vi "createfolderincrementing.vi"(8 "error in (no error)":errorcluster, 10 "Base path":path=path "bttt", 11 "Folder Name":string) -> (0 "error out":errorcluster, 3 "created path":path)   [LabVIEW 2017]
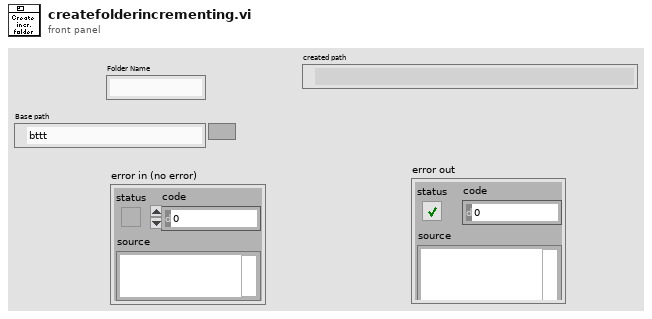
[diagram p1: front panel]
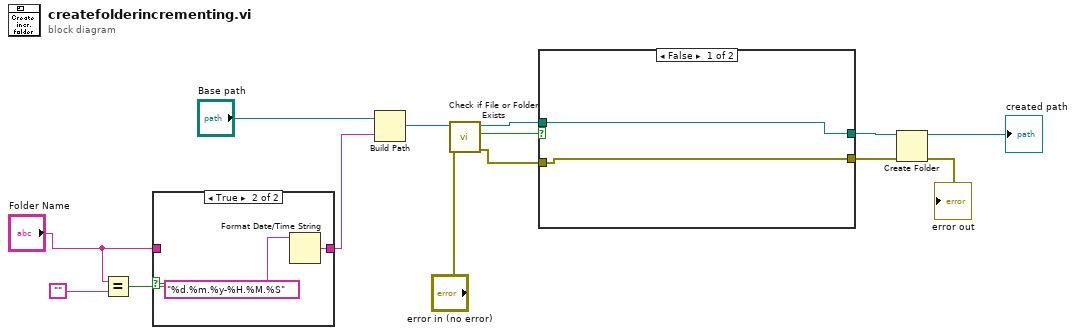
[diagram p0: block diagram]
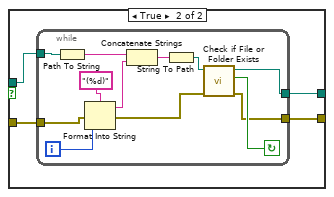
[diagram p3: hidden frame]
diagram:
  n1 = Equal?(x="Folder Name", y="") -> (x = y?=w4:bool)
  n2 = case shown="True" w4 {
    tunnel: [w15 w17] -> w3
    tunnel: "Folder Name" -> [w15 _]
    frame False {
    }
    frame True {
      n3 = Format Date/Time String(time format string (%c)="%d.%m.%y-%H.%M.%S") -> (date/time string=w17:string)  [unwired: 2 in]
    }
  }
  n4 = Build Path(base path="Base path", name or relative path=w3) -> (appended path=w14:path)
  n5 = call <vilib>:"Check if File or Folder Exists.vi"("error in (no error)"="error in (no error)", "path"=w14) -> ("error out"=w8:errorcluster, "file or folder exists?"=w13:bool, "dup path"=w11:path)  [unwired: 7 in]
  n6 = case shown="False" w13 {
    tunnel: [w19 w22] -> w12
    tunnel: w11 -> [w19 w23]
    tunnel: [w18 w21] -> w9
    tunnel: w8 -> [w18 w20]
    frame False {
    }
    frame True {
      n7 = while {
        tunnel: w23 -> [w28]
        tunnel: [w32] -> w22
        tunnel: [w31] -> w21
        tunnel: w20 -> [w29]
        i -> [w34]
        stop <- w35 continue-if-true
        n8 = Path To String(path=w28) -> (string=w27:string)
        n9 = Format Into String(format string="(%d)", error in=w29, w34) -> (resulting string=w26:string, error out=w30:errorcluster)  [unwired: 1 in]
        n10 = Concatenate Strings(w27, w26) -> (w25:string)
        n11 = String To Path(string=w25) -> (path=w24:path)
        n12 = call <vilib>:"Check if File or Folder Exists.vi"("error in (no error)"=w30, "path"=w24) -> ("error out"=w31:errorcluster, "file or folder exists?"=w35:bool, "dup path"=w32:path)  [unwired: 7 in]
      }
    }
  }
  n13 = Create Folder(path (use dialog)=w12, error in=w9) -> (created path=→"created path":path, error out=→"error out":errorcluster)  [unwired: 1 in, 1 out]
